vi "SAPI Check Speak Status SubVI.vi"(8 "error in (no error)":errorcluster, 11 "speech object references":T1) -> (0 "error out":errorcluster, 2 "Status (T: Done)":bool, 3 "speech object references (out)":T1)   [LabVIEW 2009, in "SAPI.TTS.lvlib"]
doc: "Check the status of the SAPI voice object and report whether it is done speaking to the output device."
uses:
  SAPI.TTS.lvlib
  Controls/Speech object references.ctl
panel:
  # "Check the status of the SAPI voice\nobject and report whether it is done\nspeaking to the output device."
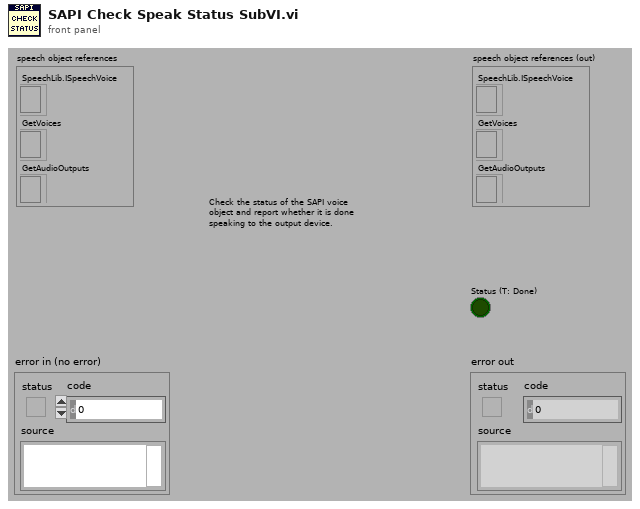
[diagram p1: front panel]
types:
  T1 = typedef "SAPI.TTS.lvlib/Speech object references.ctl" = cluster{"SpeechLib.ISpeechVoice":refnum<k7>, "GetVoices":refnum<k7>, "GetAudioOutputs":refnum<k7>}
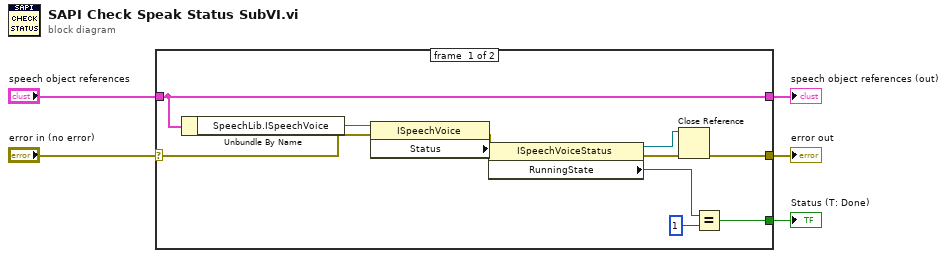
[diagram p0: block diagram]
diagram:
  n1 = case shown="No Error" "error in (no error)" {
    selector: "error in (no error)" -> [w6 w18]
    tunnel: [w11 w18] -> w4
    tunnel: "speech object references" -> [w15 w17]
    tunnel: [w15 w17] -> w1
    tunnel: [w8 _] -> w2
    frame #0 {
      n2 = Unbundle By Name(w15) -> ("SpeechLib.ISpeechVoice"=w16:refnum<k7>)
      n3 = property class="ISpeechVoice"(reference=w16, error in=w6) -> (error out=w7:errorcluster, "Status"=w14:refnum<k7>)  [unwired: 1 out]
      n4 = property class="ISpeechVoiceStatus"(reference=w14, error in=w7) -> (reference out=w13:refnum<k7>, error out=w12:errorcluster, "RunningState"=w10:i32)
      n5 = Close Reference(reference=w13, error in (no error)=w12) -> (error out=w11:errorcluster)
      n6 = Equal?(x=w10, y=1) -> (x = y?=w8:bool)
    }
    frame #1 {
    }
  }
  "error out" <- w4
  "Status (T: Done)" <- w2
  "speech object references (out)" <- w1
